vi "RTS Macro Find Transisition.vi"(7 "Time":dbl[](array[numeric])=array[53894 elements] format="%<%H:%M:%S>t", 8 "Error In":errorcluster, 10 "Input Pulse Train":dbl[](array[numeric])) -> (0 "Error Out":errorcluster, 1 "Transisition Index":i32, 2 "Output Dataset":dbl[](array[numeric]), 5 "Transistion Timestamp":dbl format="%<%H:%M:%S>t")   [LabVIEW 2016]
uses:
  <vilib>/ptbypt/NI_PtbyPt.lvlib
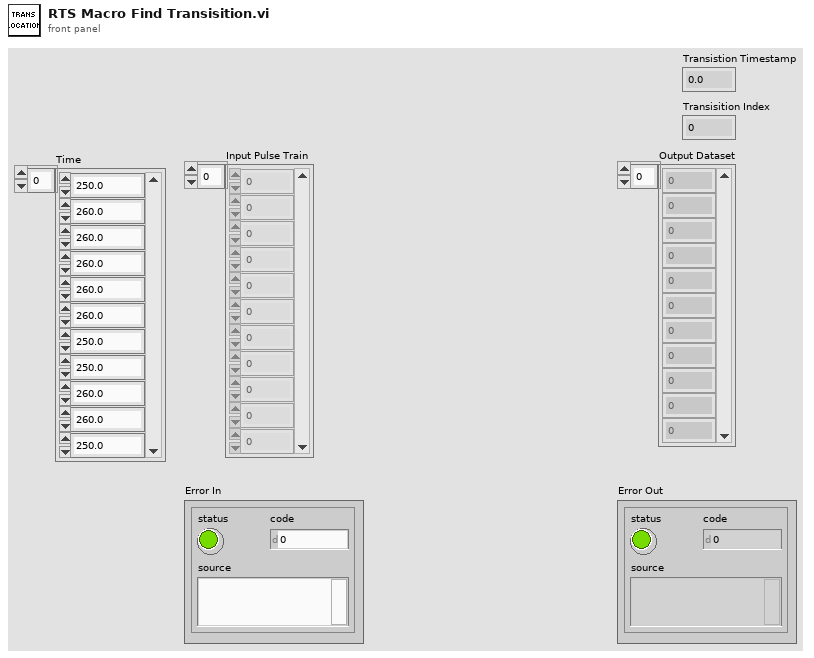
[diagram p1: front panel]
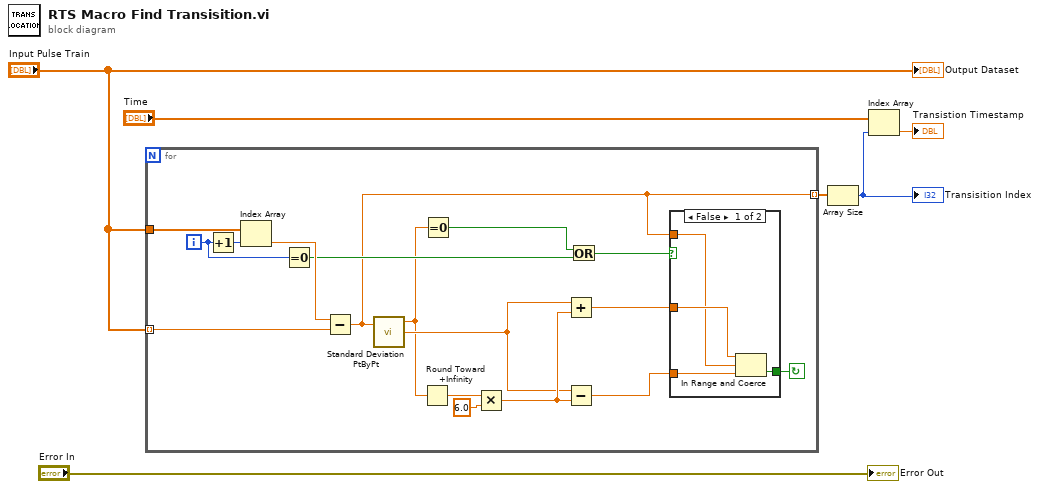
[diagram p0: block diagram]
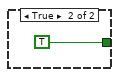
[diagram p2: hidden frame]
diagram:
  n1 = for {
    tunnel: "Input Pulse Train" -> [w23] mode=indexing
    tunnel: [w12] -> w6 mode=indexing
    tunnel: "Input Pulse Train" -> [w22]
    i -> [w16]
    stop <- w17 continue-if-true
    n2 = Increment(x=w16) -> (x+1=w21:i32)
    n3 = Index Array(array=w22, index=w21) -> (element=w20:dbl)
    n4 = Equal To 0?(x=w16) -> (x = 0?=w14:bool)
    n5 = Subtract(x=w20, y=w23) -> (x-y=w12:dbl)
    n6 = call <vilib>:"Standard Deviation PtByPt.vi"("x"=w12) -> ("standard deviation"=w11:dbl, "mean"=w15:dbl)  [unwired: 2 in, 1 out]
    n7 = Round Toward +Infinity(x=w11) -> (ceil(x): smallest int >= x=w10:dbl)
    n8 = Equal To 0?(x=w11) -> (x = 0?=w9:bool)
    n9 = Multiply(x=w10, y=6.0) -> (x*y=w18:dbl)
    n10 = Add(x=w15, y=w18) -> (x+y=w7:dbl)
    n11 = Subtract(x=w15, y=w18) -> (x-y=w8:dbl)
    n12 = Or(x=w9, y=w14) -> (x .or. y?=w13:bool)
    n13 = case shown="False" w13 {
      tunnel: w7 -> [w27 _]
      tunnel: w8 -> [w26 _]
      tunnel: w12 -> [w25 _]
      tunnel: [w24 TRUE] -> w17
      frame False {
        n14 = In Range and Coerce(upper limit=w27, x=w25, lower limit=w26) -> (In Range?=w24:bool)  [unwired: 1 out]
      }
      frame True {
      }
    }
  }
  n15 = Array Size(array=w6) -> (size(s)=w4:i32)
  "Transisition Index" <- w4
  n16 = Index Array(array="Time", index=w4) -> (element=→"Transistion Timestamp":dbl)
  "Error Out" <- "Error In"
  "Output Dataset" <- "Input Pulse Train"
